vi "Center Mass (Sub VI).vi"(3 "Z4":dbl, 4 "Z3":dbl, 5 "Z2":dbl, 6 "Z1":dbl) -> (0 "XY Graph":cluster{dbl[], dbl[]}(graph))   [LabVIEW 2012]
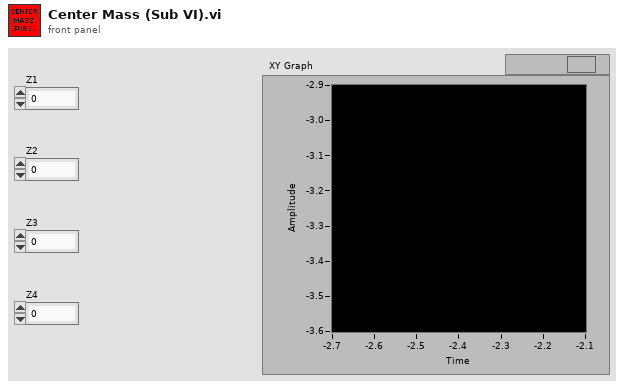
[diagram p1: front panel]
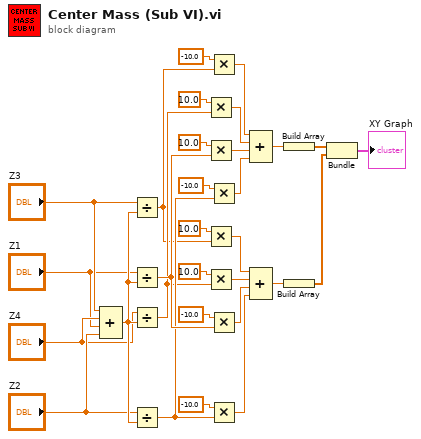
[diagram p0: block diagram]
diagram:
  n1 = Compound Arithmetic op=ADD("Z3", "Z4", "Z1", "Z2") -> (w30:dbl)
  n2 = Divide(x="Z3", y=w30) -> (x/y=w26:dbl)
  n3 = Divide(x="Z1", y=w30) -> (x/y=w29:dbl)
  n4 = Divide(x="Z4", y=w30) -> (x/y=w27:dbl)
  n5 = Divide(x="Z2", y=w30) -> (x/y=w28:dbl)
  n6 = Multiply(x=10.0, y=w27) -> (x*y=w16:dbl)
  n7 = Multiply(x=10.0, y=w29) -> (x*y=w15:dbl)
  n8 = Multiply(x=10.0, y=w26) -> (x*y=w13:dbl)
  n9 = Multiply(x=10.0, y=w27) -> (x*y=w12:dbl)
  n10 = Multiply(x=-10.0, y=w26) -> (x*y=w17:dbl)
  n11 = Multiply(x=-10.0, y=w28) -> (x*y=w14:dbl)
  n12 = Multiply(x=-10.0, y=w29) -> (x*y=w11:dbl)
  n13 = Multiply(x=-10.0, y=w28) -> (x*y=w10:dbl)
  n14 = Compound Arithmetic op=ADD(w17, w16, w15, w14) -> (w5:dbl)
  n15 = Compound Arithmetic op=ADD(w13, w12, w11, w10) -> (w6:dbl)
  n16 = Build Array(w5) -> (w8:dbl[])
  n17 = Build Array(w6) -> (w7:dbl[])
  n18 = Bundle(w8, w7) -> (→"XY Graph":cluster{dbl[], dbl[]})  [unwired: 1 in]
